vi "Show Panel Object Settings.vi"(8 "Error In":errorcluster, 11 "Pane Relief Main UI in":refnum<class "Pane Relief Main UI.lvclass">) -> (0 "Error Out":errorcluster, 3 "Pane Relief Main UI out":refnum<class "Pane Relief Main UI.lvclass">)   [LabVIEW 2018, in "Pane Relief Main UI.lvlib" / "Pane Relief Main UI.lvclass"]
uses:
  <resource>/dialog/QuickDrop/plugins/PaneRelief/Classes/Pane Relief Main UI/Pane Relief Main UI/Pane Relief Main UI.lvclass
  <resource>/dialog/QuickDrop/plugins/PaneRelief/Classes/Panel Object/Panel Object.lvclass
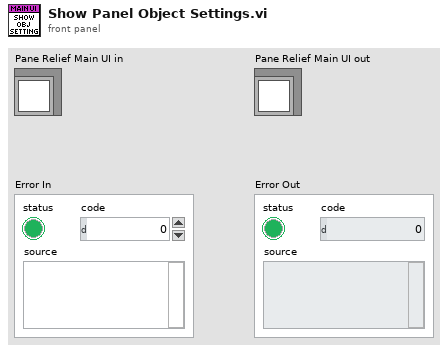
[diagram p1: front panel]
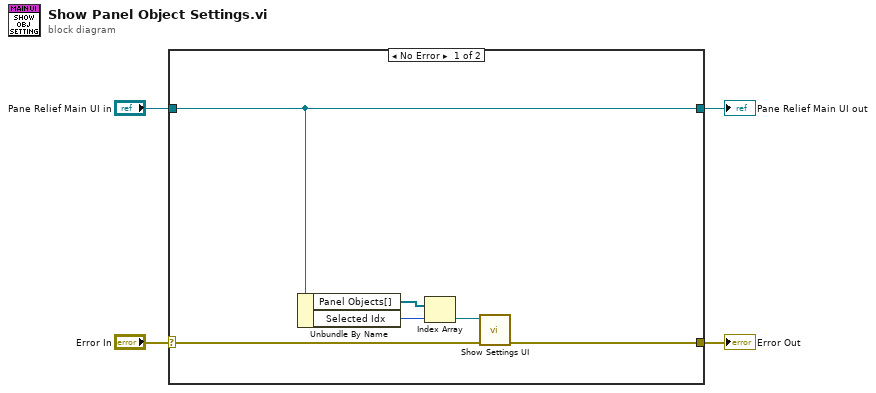
[diagram p0: block diagram]
diagram:
  n1 = case shown="No Error" "Error In" {
    selector: "Error In" -> [w6 w12]
    tunnel: [w5 w12] -> w1
    tunnel: [w7 w11] -> w3
    tunnel: "Pane Relief Main UI in" -> [w7 w11]
    frame No Error {
      n2 = Unbundle By Name(w7) -> ("Panel Objects[]"=w10:refnum<class "Panel Object.lvclass">[], "Selected Idx"=w9:i32)
      n3 = Index Array(array=w10, index=w9) -> (element=w8:refnum<class "Panel Object.lvclass">)
      n4 = call-dynamic "Show Settings UI.vi"("Error In"=w6, "Panel Object in"=w8) -> ("Error Out"=w5:errorcluster)  [unwired: 8 in, 1 out]
    }
    frame Error {
    }
  }
  "Pane Relief Main UI out" <- w3
  "Error Out" <- w1
